vi "Package Must Exist.vi"(8 "error in (no error)":errorcluster, 11 "AddAction in":refnum<class "AddAction.lvclass">) -> (0 "error out":errorcluster, 2 "Pkg Must Exist":bool, 3 "AddAction out":refnum<class "AddAction.lvclass">)   [LabVIEW 2020, in "GPackTools.lvlib" / "AddAction.lvclass"]
uses:
  AddAction.lvclass
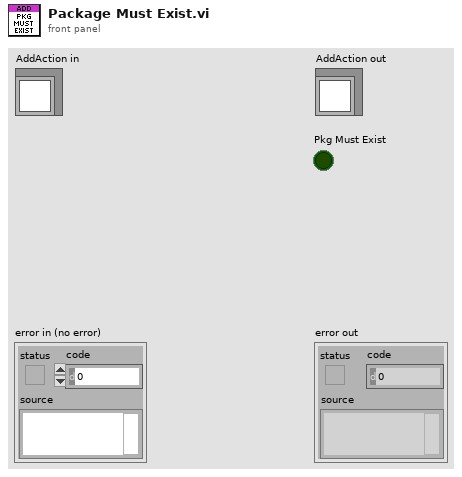
[diagram p1: front panel]
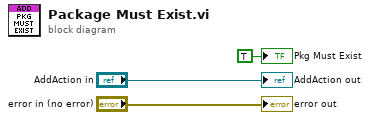
[diagram p0: block diagram]
diagram:
  "error out" <- "error in (no error)"
  "AddAction out" <- "AddAction in"
  "Pkg Must Exist" <- TRUE ("Pkg Must Exist")
